vi "test Data Width 1 to 64.vi"(8 "error in (no error)":errorcluster, 11 "TestCase in":refnum<class "BCD.lvclass">) -> (0 "error out":errorcluster, 3 "TestCase out":refnum<class "BCD.lvclass">)   [LabVIEW 2020, in "BCD.lvclass"]
uses:
  BCD.lvclass
  080c8e86-f0ef-40bb-bb78-ec3bfa871640.vi
  080c8e86-f0ef-40bb-bb78-ec3bfa871640.vi/a7fcce85-1f75-4572-aeaa-ddfd463a7c5f.vi
  BCD Decode Integer.vi/9a65bfc0-0d77-4ef3-ab58-63df1e1caa90.vi
  <vilib>/addons/_JKI Toolkits/VI Tester/TestCase.llb/TestCase.lvclass
  Encoding and Decoding.lvlib
  C:/Program Files (x86)/National Instruments/LabVIEW 2020/vi.lib/addons/_JKI Toolkits/VI Tester/TestCase.llb/TestCase.lvclass
panel:
  out "BCD encoded value":bool[](array[boolean])
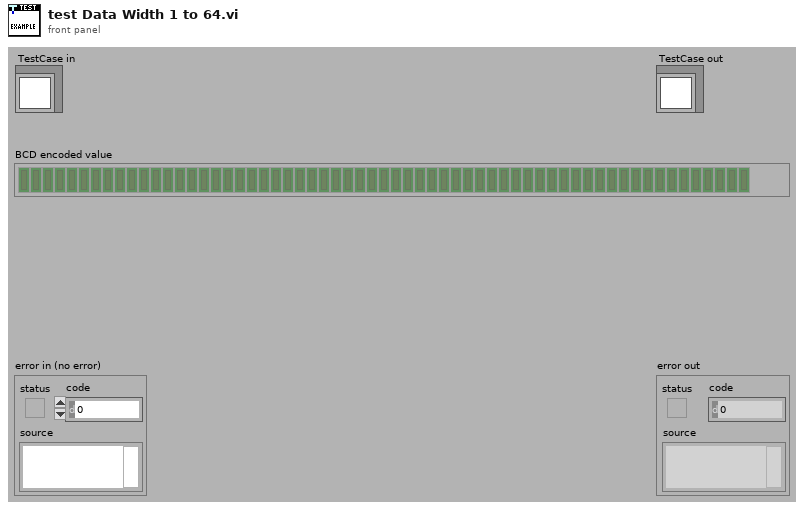
[diagram p1: front panel]
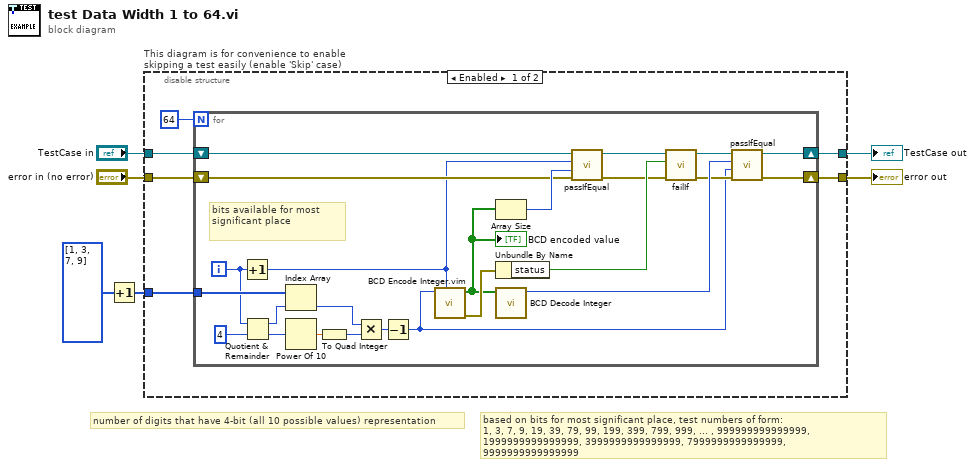
[diagram p0: block diagram]
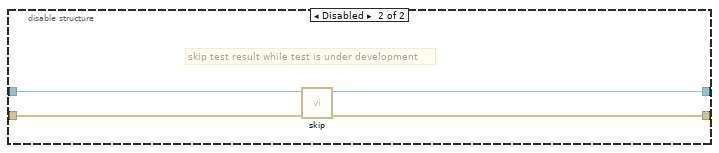
[diagram p2: hidden frame]
diagram:
  # "based on bits for most significant place, test numbers of form:\n1, 3, 7, 9, 19, 39, 79, 99, 199, 399, 799, 999, ... , 999999999999999, \n1999999999999999, 3999999999999999, 7999999999999999, 9999999999999999"
  # "number of digits that have 4-bit (all 10 possible values) representation"
  n1 = Increment(x=i64[] [1, 3, 7, 9]) -> (x+1=w1:i64[])
  n2 = disable-structure "This diagram is for convenience to enable skipping a test easily (enable 'Skip' case)" shown="Enabled" {
    disable-tunnel: "TestCase in" -> [w12 w40]
    disable-tunnel: [w10 w38] -> w3
    disable-tunnel: [w9 w39] -> w5
    disable-tunnel: "error in (no error)" -> [w11 w37]
    disable-tunnel: w1 -> [w7 _]
    frame Enabled {
      n3 = for {
        N: 64 -> [_]
        shift-right: [w24] -> w10
        shift-left: w12 -> [w31]
        shift-right: [w25] -> w9
        shift-left: w11 -> [w30]
        tunnel: w7 -> [w16]
        i -> [w15]
        # "bits available for most significant place"
        n4 = Increment(x=w15) -> (x+1=w14:i32)
        n5 = Quotient & Remainder(x=w15, y=4) -> (x-y*floor(x/y)=w18:i32, floor(x/y)=w21:i32)
        n6 = Index Array(array=w16, index=w18) -> (element=w19:i64)
        n7 = Power Of 10(x=w21) -> (10^x=w20:dbl)
        n8 = To Quad Integer(1:w20) -> (0:w22:i64)
        n9 = Multiply(x=w19, y=w22) -> (x*y=w23:i64)
        n10 = Decrement(x=w23) -> (x-1=w13:i64)
        n11 = call "BCD Encode Integer.vim"("data size (bits)"=w14, "integer"=w13) -> ("error out"=w35:errorcluster, "BCD encoded value"=w33:bool[])  [unwired: 8 in]
        "BCD encoded value" <- w33
        n12 = Array Size(array=w33) -> (size(s)=w34:i32)
        n13 = Unbundle By Name(w35) -> ("status"=w36:bool)
        n14 = call "BCD Decode Integer.vi"("BCD encoded value"=w33) -> ("integer"=w32:i64)  [unwired: 10 in]
        n15 = call-dynamic "passIfEqual.vi"("error in (no error)"=w30, "y"=w34, "x"=w14, "TestCase in"=w31) -> ("error out"=w28:errorcluster, "TestCase out"=w29:refnum<class "BCD.lvclass">)  [unwired: 6 in]
        n16 = call-dynamic "failIf.vi"("error in (no error)"=w28, "fail"=w36, "TestCase in"=w29) -> ("error out"=w26:errorcluster, "TestCase out"=w27:refnum<class "BCD.lvclass">)  [unwired: 7 in]
        n17 = call-dynamic "passIfEqual.vi"("error in (no error)"=w26, "y"=w13, "x"=w32, "TestCase in"=w27) -> ("error out"=w25:errorcluster, "TestCase out"=w24:refnum<class "BCD.lvclass">)  [unwired: 6 in]
      }
    }
    frame Disabled {
      # "skip test result while test is under development"
      n18 = call <vilib>:"skip.vi"("error in (no error)"=w37, "TestCase in"=w40) -> ("error out"=w39:errorcluster, "TestCase out"=w38:refnum<class "BCD.lvclass">)  [unwired: 8 in]
    }
  }
  "error out" <- w5
  "TestCase out" <- w3
